vi "Write Configuration.vi"(8 "error in (no error)":errorcluster, 10 "Variant":variant, 11 "Configuration in":refnum<class "Configuration.lvclass">) -> (0 "error out":errorcluster, 3 "Configuration out":refnum<class "Configuration.lvclass">)   [LabVIEW 2019, in "Configuration.lvclass"]
uses:
  Configuration.lvclass
  Configuration.lvclass/Configuration.ctl
  <vilib>/Utility/config.llb/NI_LVConfig.lvlib
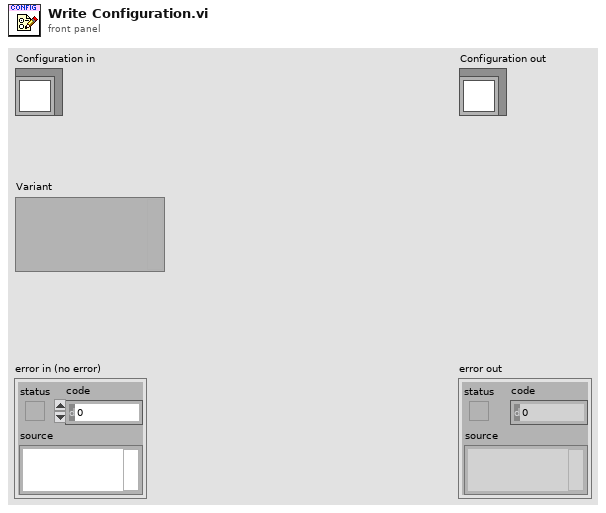
[diagram p1: front panel]
types:
  T1 = typedef "NI_LVConfig.lvlib/Config Data RefNum.ctl" = refnum<k1>
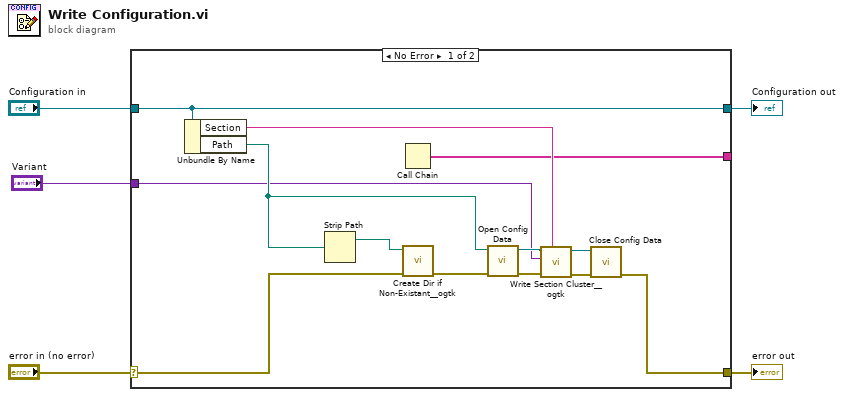
[diagram p0: block diagram]
diagram:
  n1 = case shown="No Error" "error in (no error)" {
    selector: "error in (no error)" -> [w11 w20]
    tunnel: [w14 w20] -> w4
    tunnel: [w7 w19] -> w2
    tunnel: "Configuration in" -> [w7 w19]
    tunnel: "Variant" -> [w10 _]
    tunnel: [w6 _] -> _
    frame No Error {
      n2 = Unbundle By Name(w7) -> ("Section"=w8:string, "Path"=w12:path)
      n3 = Strip Path(path=w12) -> (stripped path=w9:path)  [unwired: 1 out]
      n4 = Call Chain() -> (call chain=w6:string[])
      n5 = call <userlib>:"Create Dir if Non-Existant__ogtk.vi"("error in (no error)"=w11, "Directory Path"=w9) -> ("error out"=w13:errorcluster)  [unwired: 7 in, 2 out]
      n6 = call <vilib>:"Open Config Data.vi"("error in (no error)"=w13, "configuration file path"=w12) -> ("error out"=w18:errorcluster, "refnum"=w17:T1)  [unwired: 7 in, 1 out]
      n7 = call <userlib>:"Write Section Cluster__ogtk.vi"("section (optional)"=w8, "error in (no error)"=w18, "Section Formatted Cluster"=w10, "refnum"=w17) -> ("error out"=w16:errorcluster, "dup refnum"=w15:T1)  [unwired: 6 in]
      n8 = call <vilib>:"Close Config Data.vi"("error in (no error)"=w16, "refnum"=w15) -> ("error out"=w14:errorcluster)  [unwired: 8 in, 1 out]
    }
    frame Error {
    }
  }
  "error out" <- w4
  "Configuration out" <- w2
